vi "First Order Step Response.vi"(7 "Time constant [s]":dbl, 8 "Error In":errorcluster, 9 "Time Vector [s]":waveform(dbl), 10 "Initial Value":dbl, 11 "Final Value":dbl) -> (0 "Error Out":errorcluster, 1 "Response":waveform(dbl))   [LabVIEW 2020]
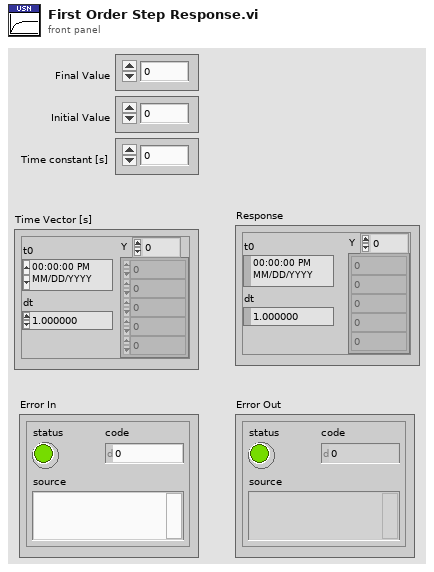
[diagram p1: front panel]
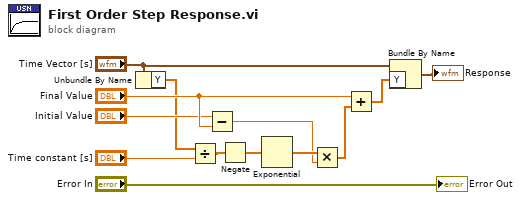
[diagram p0: block diagram]
diagram:
  n1 = Unbundle By Name("Time Vector [s]") -> ("Y"=w4:dbl[])
  n2 = Divide(x=w4, y="Time constant [s]") -> (x/y=w10:dbl[])
  n3 = Subtract(x="Initial Value", y="Final Value") -> (x-y=w6:dbl)
  n4 = Negate(x=w10) -> (-x=w11:dbl[])
  n5 = Exponential(1:w11) -> (0:w12:dbl[])
  n6 = Multiply(x=w12, y=w6) -> (x*y=w13:dbl[])
  n7 = Add(x="Final Value", y=w13) -> (x+y=w3:dbl[])
  n8 = Bundle By Name(cluster="Time Vector [s]", "Y"=w3) -> (→"Response":waveform(dbl))
  "Error Out" <- "Error In"
